vi "Configure Dialog.vi"(8 "error in (no error)":errorcluster, 11 "Configure Relays Msg.lvclass":refnum<class "Configure Relays Msg.lvclass">) -> (0 "error out":errorcluster, 2 "Ok?":bool, 3 "Configure Relays Msg.lvclass":refnum<class "Configure Relays Msg.lvclass">)   [LabVIEW 2016, in "LS218.lvlib" / "Configure Relays Msg.lvclass"]
uses:
  Configure Relays Msg.lvclass
  Configure Relays Msg.lvclass/Configure Relays Msg.ctl
panel:
  in  "Alarm Type (0:Low)":u16
  in  "Mode (0:Off)":enum16{"Off", "On", "Alarms"}(ring)
  in  "Cancel Button":bool
  in  "OK Button":bool
  in  "Input (0)":i32
  in  "Relay (0)":i32
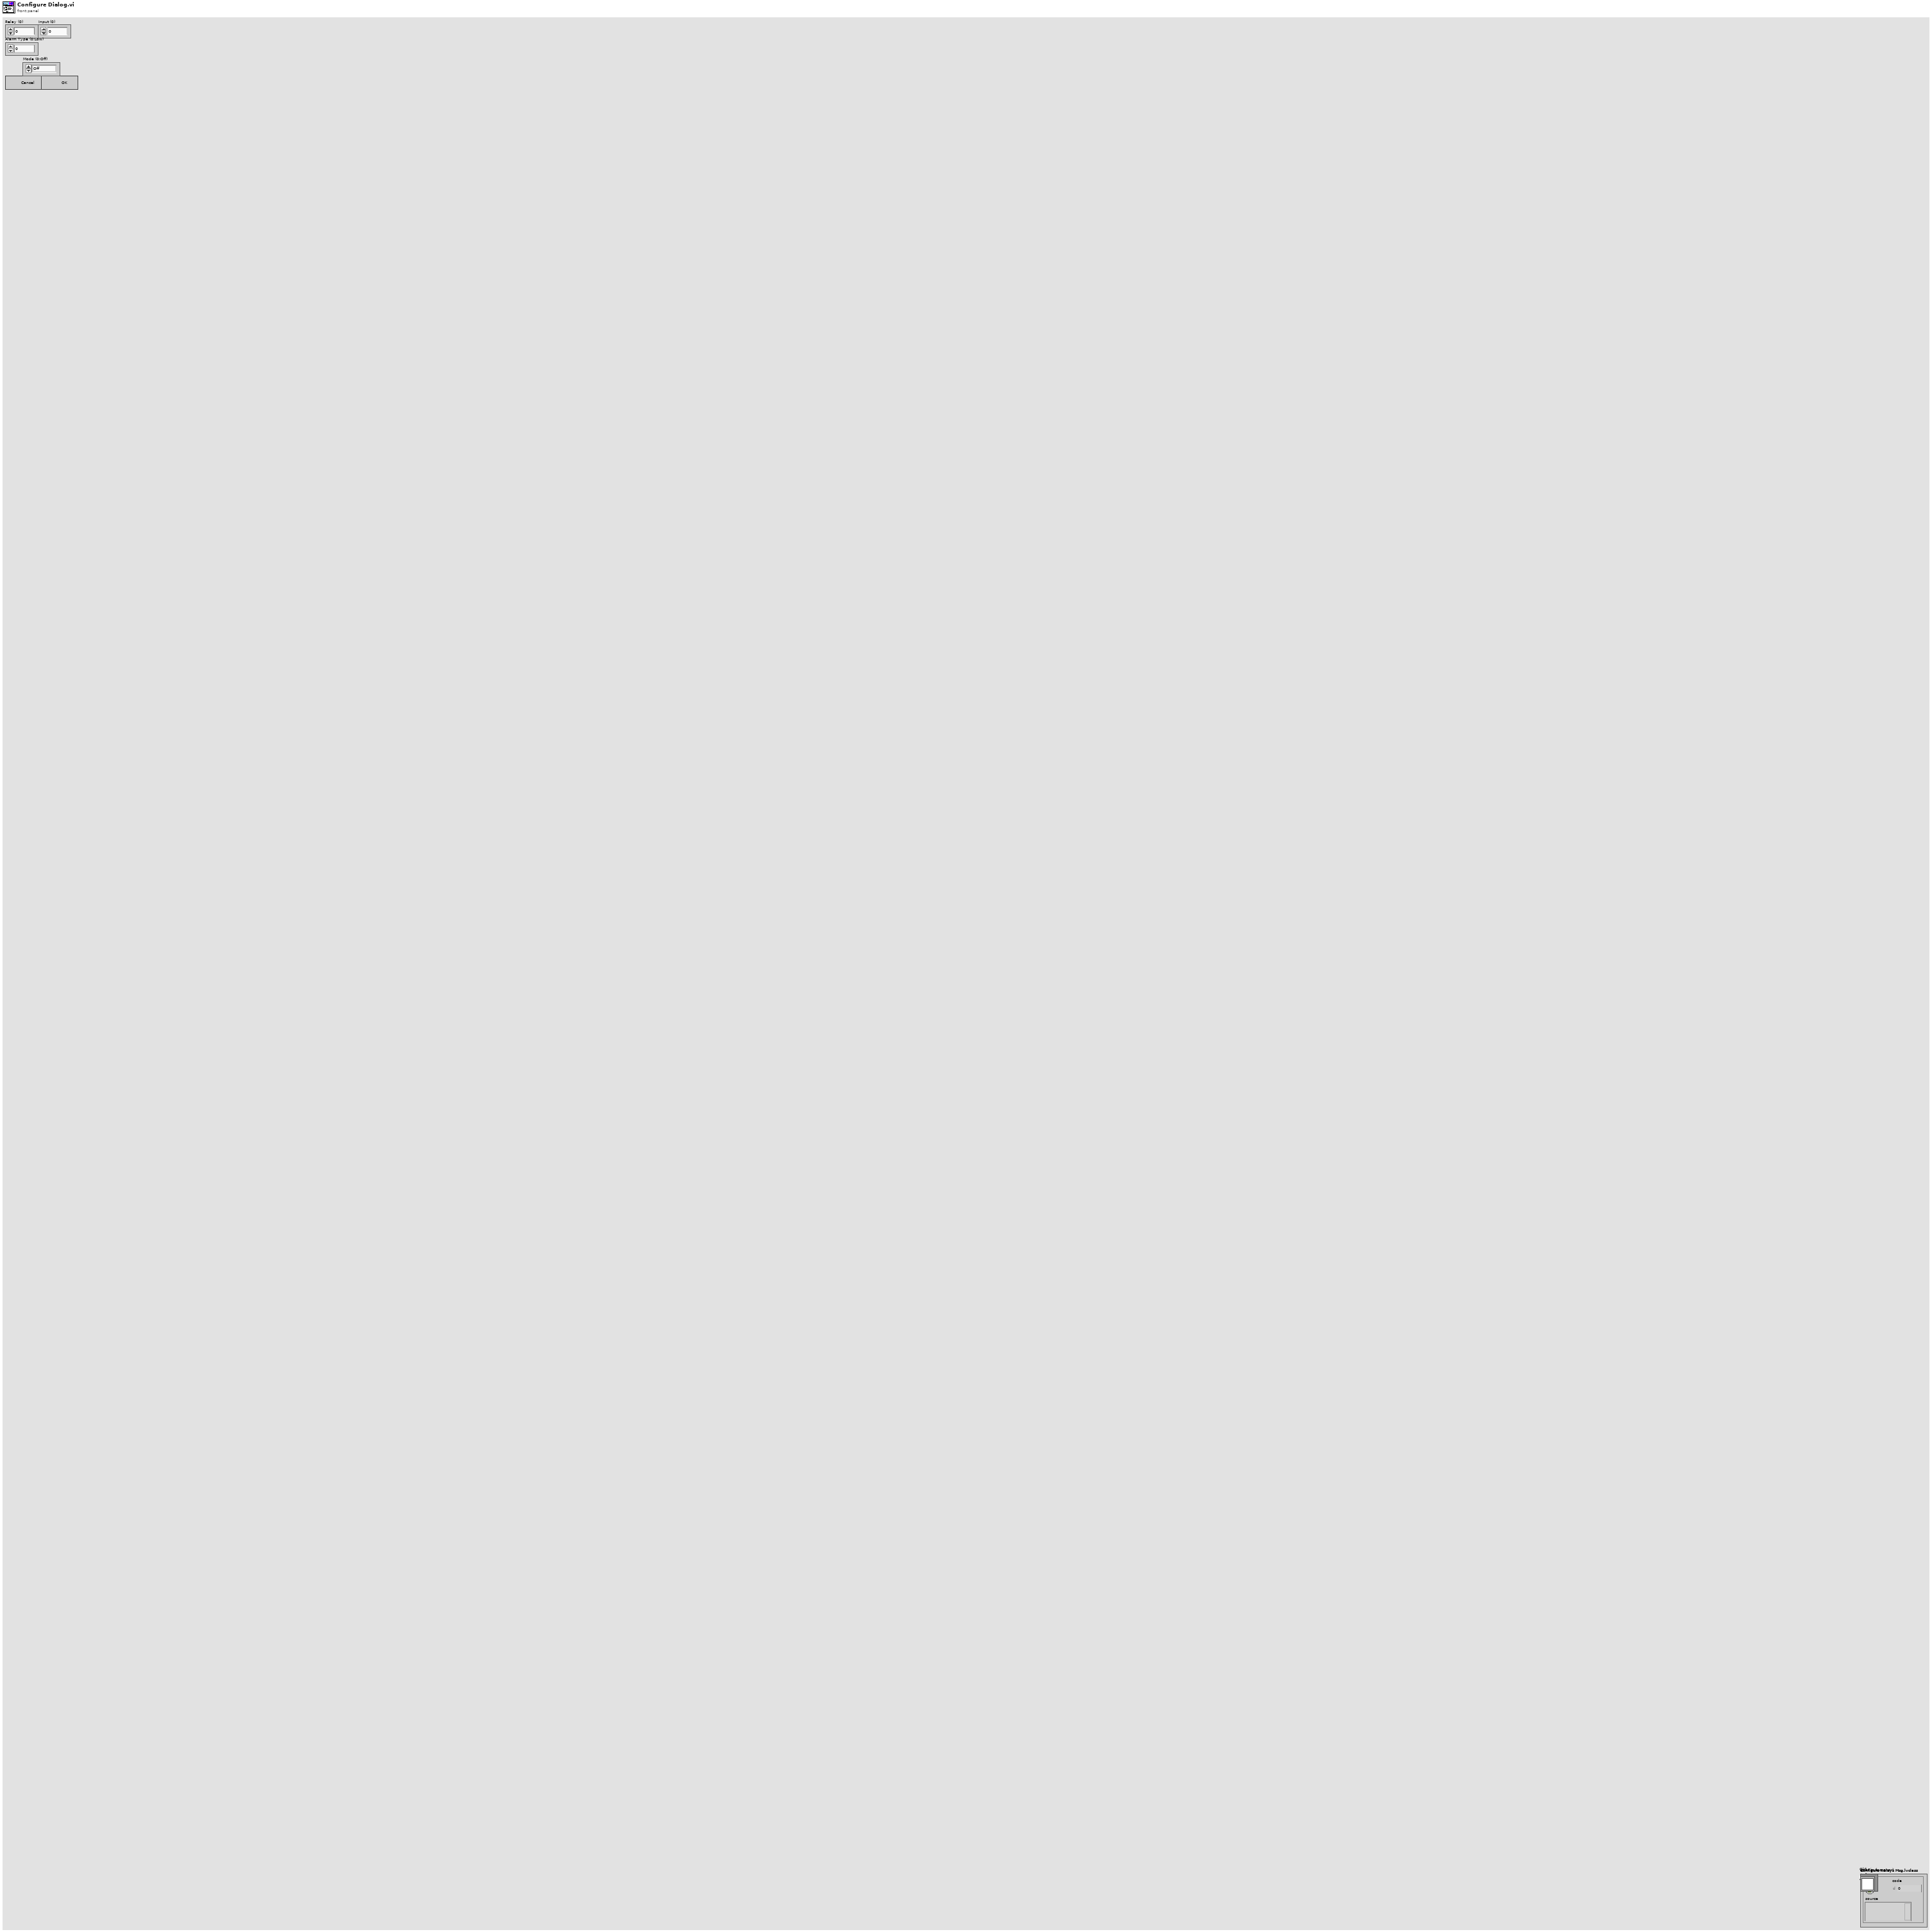
[diagram p1: front panel]
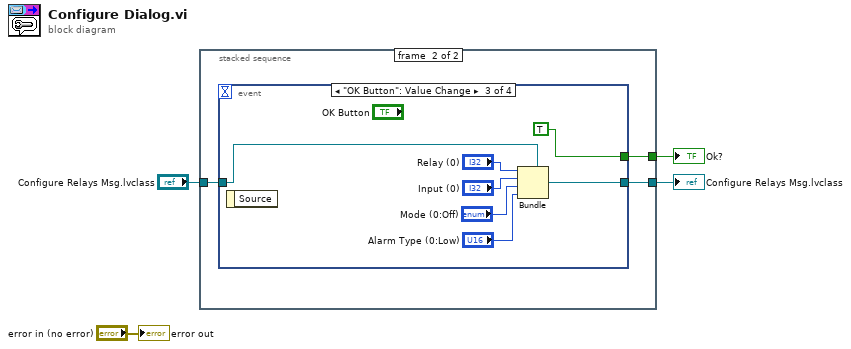
[diagram p0: block diagram]
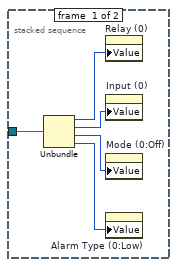
[diagram p2: hidden frame]
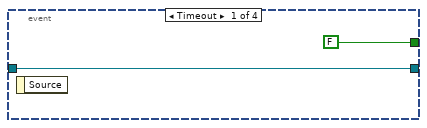
[diagram p3: hidden frame]
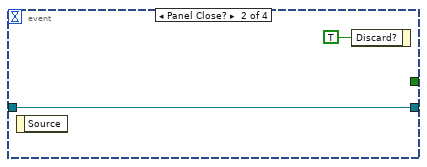
[diagram p4: hidden frame]
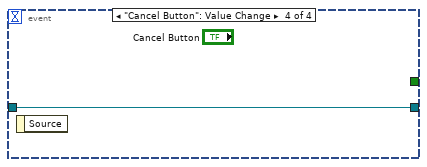
[diagram p5: hidden frame]
diagram:
  n1 = stacked-sequence {
    tunnel: [_ w12] -> w3
    tunnel: [_ w11] -> w2
    tunnel: "Configure Relays Msg.lvclass" -> [w9 w10]
    frame #0 {
      n2 = Unbundle ("Seq0Unbundler")(w9) -> (w8:i32, w7:i32, w6:enum16{"Off", "On", "Alarms"}, w5:u16)
      n3 = property on="Relay (0)" class="DigNum (strict)"("Value"=w8) -> ()  [unwired: 2 in, 2 out]
      n4 = property on="Input (0)" class="DigNum (strict)"("Value"=w7) -> ()  [unwired: 2 in, 2 out]
      n5 = property on="Mode (0:Off)" class="Enum (strict)"("Value"=w6) -> ()  [unwired: 2 in, 2 out]
      n6 = property on="Alarm Type (0:Low)" class="DigNum (strict)"("Value"=w5) -> ()  [unwired: 2 in, 2 out]
    }
    frame #1 {
      n7 = event shown="[2] \"OK Button\": Value Change" {
        selector: _ -> [_ _ _ _]
        dyn-events: _ -> [_ _ _ _]
        timeout: _ -> [_ _ _ _]
        tunnel: [w13 w15 w21 w24] -> w11
        tunnel: w10 -> [w13 w15 w23 w24]
        tunnel: [FALSE _ TRUE _] -> w12
        event Timeout {
          n8 = event-data() -> ()  [unwired: 1 in, 1 out]
        }
        event Panel Close? {
          n9 = event-data() -> ()  [unwired: 1 in, 1 out]
          n10 = event-data ("Event Filter Node")("Discard?"=TRUE) -> ()  [unwired: 1 in, 1 out]
        }
        event "OK Button": Value Change {
          n11 = event-data() -> ()  [unwired: 1 in, 1 out]
          n12 = Bundle ("Main-Bundler")(cluster=w23, "Relay (0)", "Input (0)", "Mode (0:Off)", "Alarm Type (0:Low)") -> (w21:refnum<class "Configure Relays Msg.lvclass">)
        }
        event "Cancel Button": Value Change {
          n13 = event-data() -> ()  [unwired: 1 in, 1 out]
        }
      }
    }
  }
  "Ok?" <- w3
  "Configure Relays Msg.lvclass" <- w2
  "error out" <- "error in (no error)"
